vi "TagDB-UpdateUI.vi"(7 "VIRef(Caller VI)":refnum<vi>, 8 "error in (no error)":errorcluster, 9 "force update(F)":bool, 11 "TagDB":refnum<k1>) -> (0 "error out":errorcluster, 3 "TagDB(dup)":refnum<k1>)   [LabVIEW 2017, in "TagDB.lvlib"]
uses:
  TagDB.lvlib
  fa3d7ccf-56a9-41c3-84d0-7a0938a88206.vi
  _Support/DataAccess/_NameCacher.vi
  _Support/Error/_[error50002]Invalid DataType.vi
  _Support/Error/_[error50000]Invalid DB REF.vi
  _Support/DataAccess/TagDB Ref to DVR.vi
  _Support/URL/TRIM-BOTH-SPACE.vi
  _Support/Change Detector/TagDB ChangeFlag.vi
  _Support/Error/_Build Error Cluster.vi
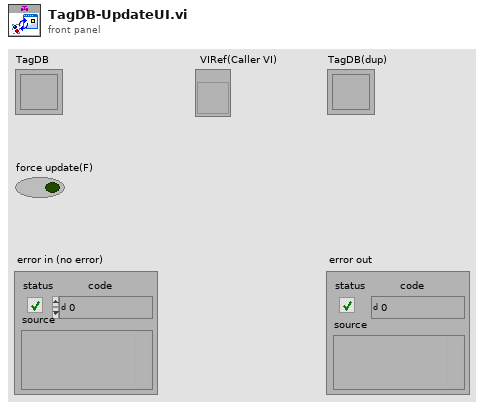
[diagram p1: front panel]
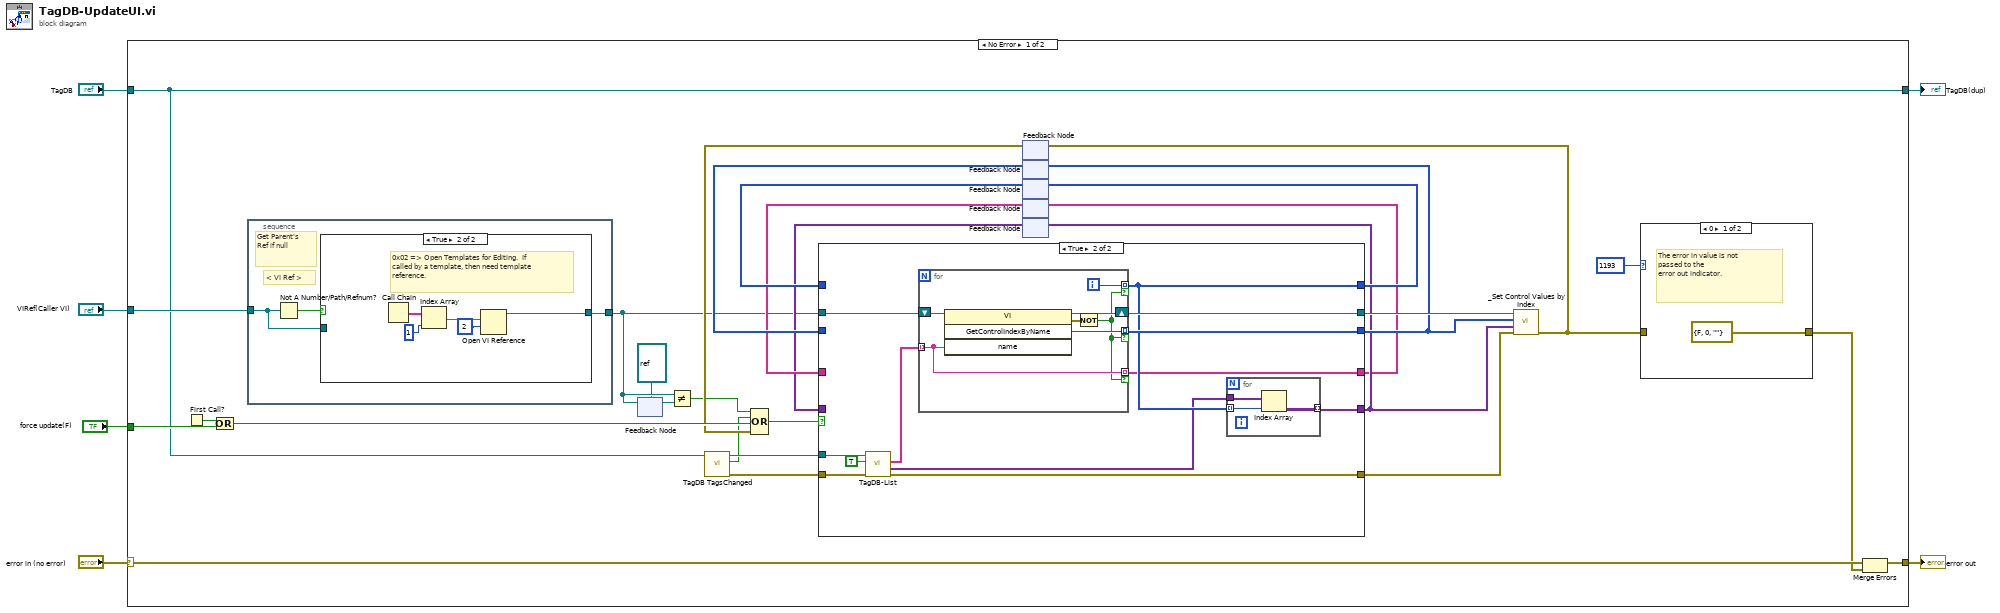
[diagram p0: block diagram]
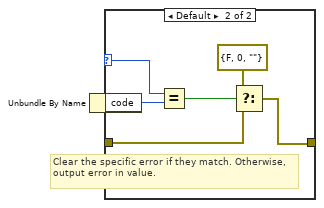
[diagram p2: hidden frame]
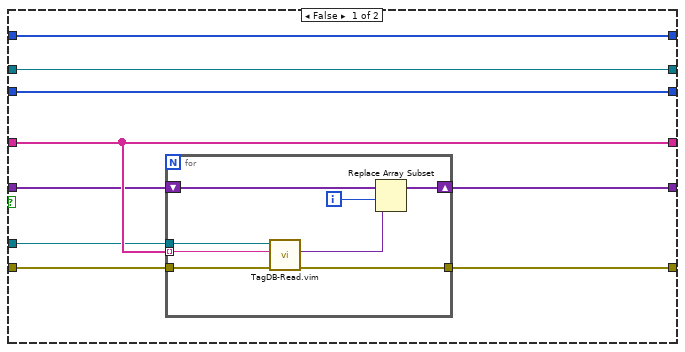
[diagram p4: hidden frame]
diagram:
  n1 = case shown="No Error" "error in (no error)" {
    selector: "error in (no error)" -> [w25 w92]
    tunnel: "VIRef(Caller VI)" -> [w35 _]
    tunnel: "force update(F)" -> [w34 _]
    tunnel: [w26 w92] -> w4
    tunnel: "TagDB" -> [w15 w91]
    tunnel: [w15 w91] -> w1
    frame No Error {
      n2 = First Call?() -> (First Call?: T/F=w31:bool)
      n3 = Or(x=w31, y=w34) -> (x .or. y?=w27:bool)
      n4 = stacked-sequence {
        tunnel: [w44] -> w11
        tunnel: w35 -> [w43]
        frame #0 {
          # "Get Parent's\nRef if null"
          # "< VI Ref >"
          n5 = Not A Number/Path/Refnum?(number/path/refnum=w43) -> (NaN/Path/Refnum?=w45:bool)
          n6 = case shown="True" w45 {
            tunnel: [w46 w51] -> w44
            tunnel: w43 -> [w46 _]
            frame False {
            }
            frame True {
              # "0x02 => Open Templates for Editing.  If called by a template, then need template reference."
              n7 = Call Chain() -> (call chain=w47:string[])
              n8 = Index Array(array=w47, index=1 ("Index")) -> (element=w49:string)
              n9 = Open VI Reference(vi path=w49, options=2) -> (vi reference=w51:refnum<vi>)  [unwired: 4 in, 1 out]
            }
          }
        }
      }
      n10 = feedback #1(refnum<vi> refnum ("VIRef(Caller VI)")) -> (w12:refnum<vi>)
      n11 = feedback-in #1(w11) -> ()
      n12 = Not Equal?(x=w11, y=w12) -> (x != y?=w7:bool)
      n13 = call "TagDB TagsChanged.vi"("DB Ref"=w15) -> ("error in (no error) (dup)"=w13:errorcluster, "item changed?"=w9:bool, "DB Ref (dup)"=w14:refnum<k1>)  [unwired: 8 in]
      n14 = feedback #2() -> (w17:errorcluster)  [unwired: 1 in]
      n15 = Compound Arithmetic op=OR(w7, w9, w27, w17) -> (w8:bool)
      n16 = feedback #3() -> (w29:i32[])  [unwired: 1 in]
      n17 = feedback #4() -> (w30:i32[])  [unwired: 1 in]
      n18 = feedback #5() -> (w24:string[])  [unwired: 1 in]
      n19 = feedback #6() -> (w21:variant[])  [unwired: 1 in]
      n20 = case shown="True" w8 {
        tunnel: [w60 w80] -> w33
        tunnel: w11 -> [w60 w79]
        tunnel: [w58 w78] -> w32
        tunnel: [w59 w77] -> w28
        tunnel: w30 -> [w59 _]
        tunnel: w29 -> [w58 _]
        tunnel: [w56 w76] -> w19
        tunnel: w24 -> [w56 _]
        tunnel: [w54 w75] -> w22
        tunnel: w14 -> [w53 w74]
        tunnel: [w57 w73] -> w23
        tunnel: w21 -> [w55 _]
        tunnel: w13 -> [w52 w69]
        frame False {
          n21 = for {
            tunnel: [w68] -> w57
            tunnel: w56 -> [w67] mode=indexing
            shift-right: [w65] -> w54
            shift-left: w55 -> [w66]
            tunnel: w53 -> [w62]
            tunnel: w52 -> [w61]
            i -> [w64]
            n22 = call "TagDB-Read.vim"("error in (no error)"=w61, "name"=w67, "TagDB"=w62) -> ("error out"=w68:errorcluster, "Value"=w63:variant)  [unwired: 3 in, 4 out]
            n23 = Replace Array Subset(array=w66, new element=w63, index=w64) -> (w65:variant[])
          }
        }
        frame True {
          n24 = call "TagDB-List.vi"("error in (no error)"=w69, "with Data?(F)"=TRUE, "TagDB"=w74) -> ("error out"=w73:errorcluster, "Data"=w72:variant[], "names"=w71:string[])  [unwired: 5 in, 1 out]
          n25 = for {
            tunnel: w71 -> [w85] mode=indexing
            tunnel: [w89] -> w78 mode=indexing if=w84
            shift-right: [w90] -> w80
            shift-left: w79 -> [w87]
            tunnel: [w86] -> w77 mode=indexing if=w84
            tunnel: [w85] -> w76 mode=indexing if=w84
            i -> [w86]
            n26 = invoke class="VI" method="GetControlIndexByName"(reference=w87, "name"=w85) -> (reference out=w90:refnum<vi>, error out=w88:errorcluster, "GetControlIndexByName"=w89:i32)  [unwired: 2 in, 1 out]
            n27 = Not(x=w88) -> (.not. x?=w84:bool)
          }
          n28 = for {
            tunnel: w77 -> [w83] mode=indexing
            tunnel: w72 -> [w82]
            tunnel: [w81] -> w75 mode=indexing
            n29 = Index Array(array=w82, index=w83) -> (element=w81:variant)
          }
        }
      }
      n30 = feedback-in #3(w32) -> ()
      n31 = feedback-in #4(w28) -> ()
      n32 = feedback-in #5(w19) -> ()
      n33 = feedback-in #6(w22) -> ()
      n34 = call "_Set Control Values by Index.vi"("error in (no error)"=w23, "data values"=w22, "control indexes"=w32, "VI Refnum"=w33) -> ("error out"=w18:errorcluster)  [unwired: 7 in]
      n35 = feedback-in #2(w18) -> ()
      n36 = case shown="0" 1193 ("specific error code to clear (0: all)") {
        selector: 1193 ("specific error code to clear (0: all)") -> [_ w41]
        tunnel: w18 -> [_ w40]
        tunnel: [errorcluster {"status"=FALSE, "code"=0, "source"=""} ("error constant") w37] -> w20
        frame 0 {
          # "The error in value is not passed to the\nerror out indicator."
        }
        frame Default {
          # "Clear the specific error if they match. Otherwise, output error in value."
          n37 = Unbundle By Name(w40) -> ("code"=w42:i32)
          n38 = Equal?(x=w41, y=w42) -> (x = y?=w38:bool)
          n39 = Select(t=errorcluster {"status"=FALSE, "code"=0, "source"=""} ("error constant"), s=w38, f=w40) -> (s? t:f=w37:errorcluster)
        }
      }
      n40 = Merge Errors(w25, w20) -> (w26:errorcluster)
    }
    frame Error {
    }
  }
  "error out" <- w4
  "TagDB(dup)" <- w1
